vi "Log Value to File.vi"(8 "error in (no error)":errorcluster, 10 "Data Record":T1, 11 "Datalogger Actor in":refnum<class "Datalogger Actor.lvclass">) -> (0 "error out":errorcluster, 3 "Datalogger Actor out":refnum<class "Datalogger Actor.lvclass">)   [LabVIEW 2018, in "Datalogger.lvlib" / "Datalogger Actor.lvclass"]
uses:
  Datalogger Actor.lvclass
  Data Record Control.ctl
  Datalogger Actor.lvclass/Datalogger Actor.ctl
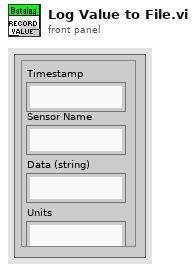
[diagram p1: front panel]
types:
  T1 = typedef "Datalogger.lvlib/Datalogger Actor.lvclass/Data Record Control.ctl" = cluster{"Timestamp":string, "Sensor Name":string, "Data (string)":string, "Units":string}
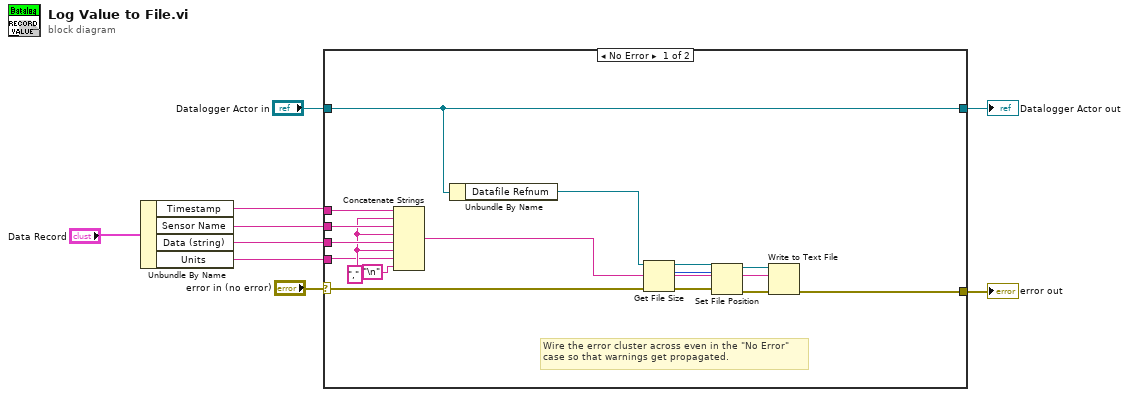
[diagram p0: block diagram]
diagram:
  n1 = Unbundle By Name("Data Record") -> ("Timestamp"=w3:string, "Sensor Name"=w2:string, "Data (string)"=w5:string, "Units"=w4:string)
  n2 = case shown="No Error" "error in (no error)" {
    selector: "error in (no error)" -> [w16 w27]
    tunnel: [w25 w27] -> w8
    tunnel: [w23 w26] -> w6
    tunnel: "Datalogger Actor in" -> [w23 w26]
    tunnel: w5 -> [w21 _]
    tunnel: w4 -> [w18 _]
    tunnel: w3 -> [w24 _]
    tunnel: w2 -> [w22 _]
    frame No Error {
      w20 = "," ("string")
      # "Wire the error cluster across even in the \"No Error\"\ncase so that warnings get propagated."
      n3 = Concatenate Strings(w24, w20, w22, w20, w21, w20, w18, "\n") -> (w10:string)
      n4 = Unbundle By Name(w23) -> ("Datafile Refnum"=w17:refnum<file>)
      n5 = Get File Size(file=w17, error in=w16) -> (refnum out=w15:refnum<file>, size (in bytes)=w13:i64, 0:w12:errorcluster)
      n6 = Set File Position(offset (in bytes) (0)=w13, refnum=w15, error in=w12) -> (refnum out=w14:refnum<file>, error out=w11:errorcluster)  [unwired: 1 in]
      n7 = Write to Text File(file (use dialog)=w14, text=w10, error in=w11) -> (error out=w25:errorcluster)  [unwired: 1 in, 2 out]
    }
    frame Error {
    }
  }
  "error out" <- w8
  "Datalogger Actor out" <- w6
